vi "SR400_standalone_test.vi"() -> ()   [LabVIEW 2013]
uses:
  Controls/SR400/Channel A/channelA_inputs.ctl
  Controls/SR400/discrim_slope.ctl
  Controls/SR400/gate_mode.ctl
  Controls/SR400/Channel A/channelA.ctl
  Controls/SR400/Channel B/inputsB.ctl
  Controls/SR400/Channel B/channelB.ctl
  Controls/SR400/Channel T/inputsT.ctl
  Controls/SR400/Channel T/channelT.ctl
  Controls/SR400/SR400.ctl
panel:
  out "Counter B Data":string[](array[string])
  out "Counter A Data":string[](array[string])
  out "error out":errorcluster
  in  "Cluster":T1={"Channel A"={"Input"=0, "A Discriminator Level (V)"=0.0, "A Discriminator Slope"=enum."Falling", "A Gate Mode"=enum."CW", "A Gate Delay (s)"=0.0, "A Gate Width (s)"=5e-09, "Scan Increment (s)"=0.0}, "Channel B"={"Input"=0, "B Discriminator Level (V)"=0.0, "B Discriminator Slope"=enum."Falling", "B Gate Mode"=enum."CW", "B Gate Delay (s)"=0.0, "B Gate Width (s)"=5e-09, "Scan Increment (s)"=0.0}, "Channel T"={"Input"=0, "Trigger Level (V)"=0.0, "Trigger Slope"=enum."Falling", "T Discriminator Slope"=enum."Falling", "T Discriminator Level (V)"=0.0, "Trigger Preset"=1.0}, "N Periods"=1.0, "At N"=enum."Stop", "Counting Mode"=enum."A,B for T Preset", "GPIB Address"="", "Dwell Time (s)"=0.002, "Port 1 Mode"=0, "Port 1 Voltage"=0.0, "Port 1 Scan Increment"=-0.5, "Port 2 Voltage"=0.0, "Port 2 Scan Increment"=0.0, "Port 2 Mode"=0, "Counter Toggle"=FALSE, "Pusleblater Settings"={"Loop Start Channel"=0.0, "Loop End Channel"=0.0, "Loop On"=FALSE}} {"Port 2 Mode" items=["Scan"=1, "Fixed"=0]; "Port 2 Scan Increment" min=-0.5 max=0.5; "Port 2 Voltage" min=-10.0 max=10.0; "Port 1 Scan Increment" min=-0.5 max=-0.5; "Port 1 Voltage" min=-10.0 max=10.0; "Port 1 Mode" items=["Scan"=1, "Fixed"=0]; "Dwell Time (s)" min=0.002 max=60.0 format="%#_6p"; "N Periods" min=1.0 max=2000.0 step=1.0; "Channel T"."Trigger Preset" min=1.0 max=900000000000.0 format="%#_1e"; "Channel T"."T Discriminator Level (V)" min=-0.3 max=0.3 format="%#_6p"; "Channel T"."Trigger Level (V)" min=-2.0 max=2.0 format="%#_6p"; "Channel T"."Input" items=["10 MHz", "Input 2", "Trig"]; "Channel B"."Scan Increment (s)" min=0.0 max=0.09992 format="%#_6p"; "Channel B"."B Gate Width (s)" min=5e-09 max=0.9992 format="%#_6p"; "Channel B"."B Gate Delay (s)" min=0.0 max=0.9992 format="%#_6p"; "Channel B"."B Discriminator Level (V)" min=-0.3 max=0.3 format="%#_6p"; "Channel B"."Input" items=["Input 2"=2, "Input 1"=1]; "Channel A"."Scan Increment (s)" min=0.0 max=0.09992 format="%#_6p"; "Channel A"."A Gate Width (s)" min=5e-09 max=0.9992 format="%#_6p"; "Channel A"."A Gate Delay (s)" min=0.0 max=0.9992 format="%#_6p"; "Channel A"."A Discriminator Level (V)" min=-0.3 max=0.3 format="%#_6p"; "Channel A"."Input" items=["Input 1", "10 MHz"]}
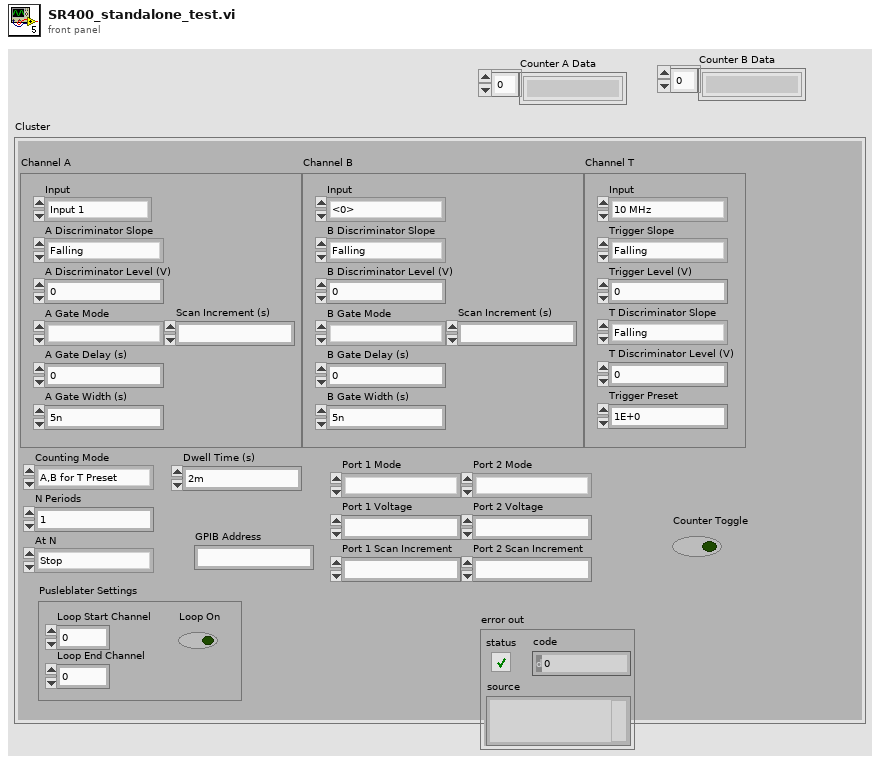
[diagram p1: front panel]
types:
  T1 = typedef "SR400.ctl" = cluster{"Channel A":T2, "Channel B":T6, "Channel T":T8, "N Periods":dbl, "At N":enum16{"Stop", "Start"}, "Counting Mode":enum16{"A,B for T Preset", "A-B for T Preset", "A+B for T Preset"}, "GPIB Address":string, "Dwell Time (s)":dbl, "Port 1 Mode":i32, "Port 1 Voltage":dbl, "Port 1 Scan Increment":dbl, "Port 2 Voltage":dbl, "Port 2 Scan Increment":dbl, "Port 2 Mode":i32, "Counter Toggle":bool, "Pusleblater Settings":cluster{"Loop Start Channel":dbl, "Loop End Channel":dbl, "Loop On":bool}}
  T2 = typedef "channelA.ctl" = cluster{"Input":T3, "A Discriminator Level (V)":dbl, "A Discriminator Slope":T4, "A Gate Mode":T5, "A Gate Delay (s)":dbl, "A Gate Width (s)":dbl, "Scan Increment (s)":dbl}
  T3 = typedef "channelA_inputs.ctl" = u16
  T4 = typedef "discrim_slope.ctl" = enum16{"Rising", "Falling"}
  T5 = typedef "gate_mode.ctl" = enum16{"CW", "Fixed", "Scan"}
  T6 = typedef "channelB.ctl" = cluster{"Input":T7, "B Discriminator Level (V)":dbl, "B Discriminator Slope":T4, "B Gate Mode":T5, "B Gate Delay (s)":dbl, "B Gate Width (s)":dbl, "Scan Increment (s)":dbl}
  T7 = typedef "inputsB.ctl" = u16
  T8 = typedef "channelT.ctl" = cluster{"Input":T9, "Trigger Level (V)":dbl, "Trigger Slope":T4, "T Discriminator Slope":T4, "T Discriminator Level (V)":dbl, "Trigger Preset":dbl}
  T9 = typedef "inputsT.ctl" = u16
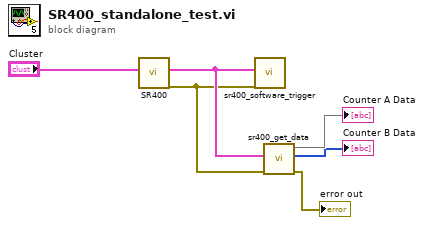
[diagram p0: block diagram]
diagram:
  n1 = call "SR400.vi"("Settings In"="Cluster") -> ("error out"=w1:errorcluster, "Settings Out"=w2:T1)  [unwired: 9 in]
  n2 = call "sr400_software_trigger.vi"("error in (no error)"=w1, "Settings In"=w2) -> ()  [unwired: 8 in, 2 out]
  n3 = call "sr400_get_data.vi"("error in (no error)"=w1, "Settings In"=w2) -> ("error out"=→"error out":errorcluster, "Counter A Data"=→"Counter B Data":i32[], 3:→"Counter A Data")  [unwired: 6 in, 1 out]
